vi "Get Array Element at Index - Object.vi"(8 "error in (no error)":errorcluster, 10 "Index":i32, 11 "YAML Parser in":refnum<class "YAML Parser.lvclass">) -> (0 "error out":errorcluster, 1 "Is Null?":bool, 2 "Object":refnum<class "YAML Parser.lvclass">, 3 "YAML Parser out":refnum<class "YAML Parser.lvclass">)   [LabVIEW 2015, in "YAML Parser.lvclass"]
uses:
  YAML Parser.lvclass
  YAML Parser.lvclass/YAML Parser.ctl
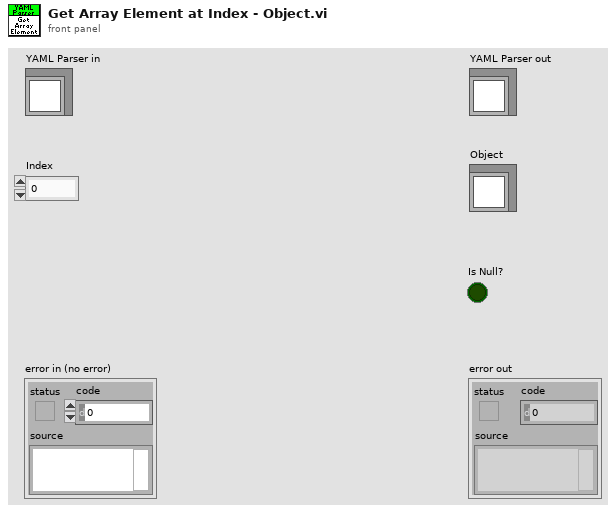
[diagram p1: front panel]
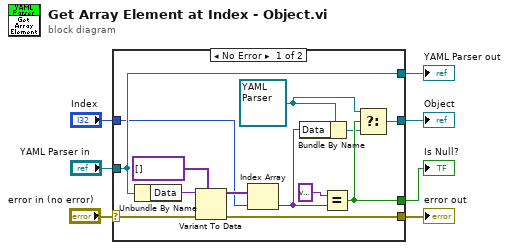
[diagram p0: block diagram]
diagram:
  n1 = case shown="No Error" "error in (no error)" {
    selector: "error in (no error)" -> [w20 w22]
    tunnel: [w18 w22] -> w6
    tunnel: [w19 w21] -> w4
    tunnel: "YAML Parser in" -> [w19 w21]
    tunnel: "Index" -> [w11 _]
    tunnel: [w15 _] -> w1
    tunnel: [w16 _] -> w2
    frame No Error {
      w8 = refnum<class "YAML Parser.lvclass"> refnum ("Object")
      n2 = Unbundle By Name(w19) -> ("Data"=w14:variant)
      n3 = Variant To Data(error in=w20, type=variant[] [], Variant=w14) -> (data=w12:variant[], error out=w18:errorcluster)
      n4 = Index Array(array=w12, index=w11) -> (element=w10:variant)
      n5 = Bundle By Name(cluster=w8, "Data"=w10) -> (w9:refnum<class "YAML Parser.lvclass">)
      n6 = Equal?(x=variant, y=w10) -> (x = y?=w16:bool)
      n7 = Select(t=w8, s=w16, f=w9) -> (s? t:f=w15:refnum<class "YAML Parser.lvclass">)
    }
    frame Error {
    }
  }
  "error out" <- w6
  "YAML Parser out" <- w4
  "Is Null?" <- w2
  "Object" <- w1
